vi "WindowHasSurface.vi"(8 "No Error":errorcluster, 11 "Window [SDL_Window *]":i64 format="%.0x") -> (0 "Error Out":errorcluster, 3 "Has Surface?":bool)   [LabVIEW 2024, in "SDL3.lvlib" / "Video.lvlib"]
doc: "<B>Summary</B>\nReturn whether the window has a surface associated with it."
uses:
  Video.lvlib
  Lib/SDL3-32.dll
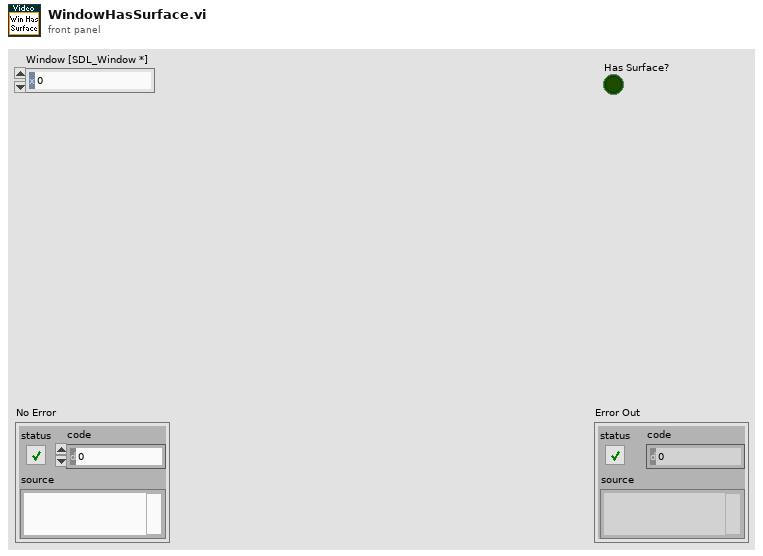
[diagram p1: front panel]
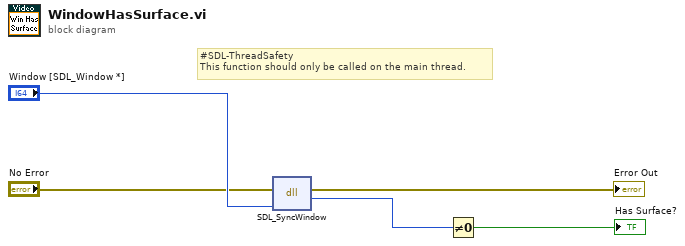
[diagram p0: block diagram]
diagram:
  # "#SDL-ThreadSafety\nThis function should only be called on the main thread."
  n1 = dll-call lib="C:/Users/Thomas/Documents/Projects/LV-SDL3/Lib/SDL3-*.*" fn="SDL_SyncWindow"(error in="No Error", "window"="Window [SDL_Window *]") -> (error out=→"Error Out":errorcluster, "return type"=w2:i32)  [unwired: 3 in, 1 out]
  n2 = Not Equal To 0?(x=w2) -> (x != 0?=→"Has Surface?":bool)
